vi "Creat config.vi"(11 "Refnum in":T1) -> ()   [LabVIEW 2017]
uses:
  <vilib>/Utility/config.llb/Config Data RefNum.ctl
  <vilib>/Utility/config.llb/Write Key (String).vi
  <vilib>/Utility/config.llb/NI_LVConfig.lvlib
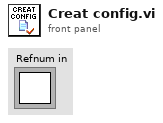
[diagram p1: front panel]
types:
  T1 = typedef "NI_LVConfig.lvlib/Config Data RefNum.ctl" = refnum<k1>
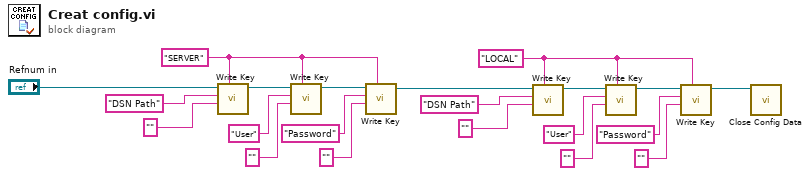
[diagram p0: block diagram]
diagram:
  w5 = "LOCAL" ("section")
  w19 = "SERVER" ("section")
  n1 = call-poly <vilib>:"Write Key.vi"("section"=w19, "value"="" ("key"), "key"="DSN Path", "refnum"="Refnum in") -> ("refnum out"=w15:T1)  [unwired: 5 in, 2 out]
  n2 = call-poly <vilib>:"Write Key.vi"("section"=w19, "value"="" ("key"), "key"="User", "refnum"=w15) -> ("refnum out"=w18:T1)  [unwired: 5 in, 2 out]
  n3 = call-poly <vilib>:"Write Key.vi"("section"=w19, "value"="" ("key"), "key"="Password", "refnum"=w18) -> ("refnum out"=w2:T1)  [unwired: 5 in, 2 out]
  n4 = call-poly <vilib>:"Write Key.vi"("section"=w5, "value"="" ("key"), "key"="DSN Path", "refnum"=w2) -> ("refnum out"=w9:T1)  [unwired: 5 in, 2 out]
  n5 = call-poly <vilib>:"Write Key.vi"("section"=w5, "value"="" ("key"), "key"="User", "refnum"=w9) -> ("refnum out"=w6:T1)  [unwired: 5 in, 2 out]
  n6 = call-poly <vilib>:"Write Key.vi"("section"=w5, "value"="" ("key"), "key"="Password", "refnum"=w6) -> ("refnum out"=w1:T1)  [unwired: 5 in, 2 out]
  n7 = call <vilib>:"Close Config Data.vi"("refnum"=w1) -> ()  [unwired: 9 in, 2 out]
